vi "WaitForSpecificCommResponse.vi"(4 "CMD sent":string, 6 "Check period (msecs)":dbl=30.0, 7 "Display err mess?":bool=TRUE, 8 "error in (no error)":errorcluster, 9 "Timeout (mSecs)":dbl=3000.0, 10 "Wait for":string, 11 "VISA Refnum in":refnum<visa-resource-name>="COM30") -> (0 "error out":errorcluster, 1 "timeout":bool, 2 "Response":string, 3 "VISA Refnum out":refnum<visa-resource-name>, 5 "Elapsed secs":dbl)   [LabVIEW 2024]
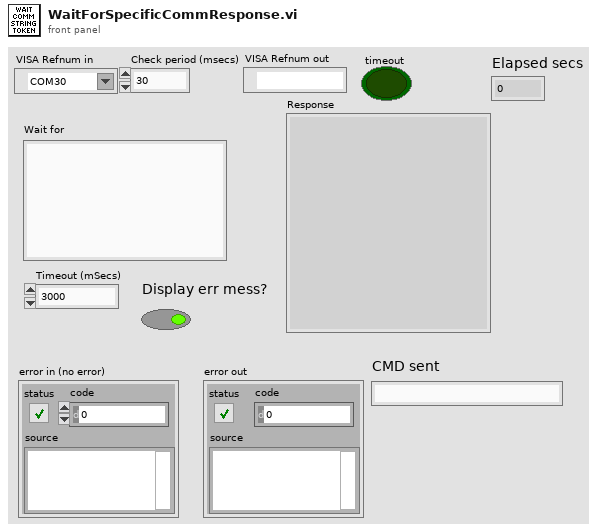
[diagram p1: front panel]
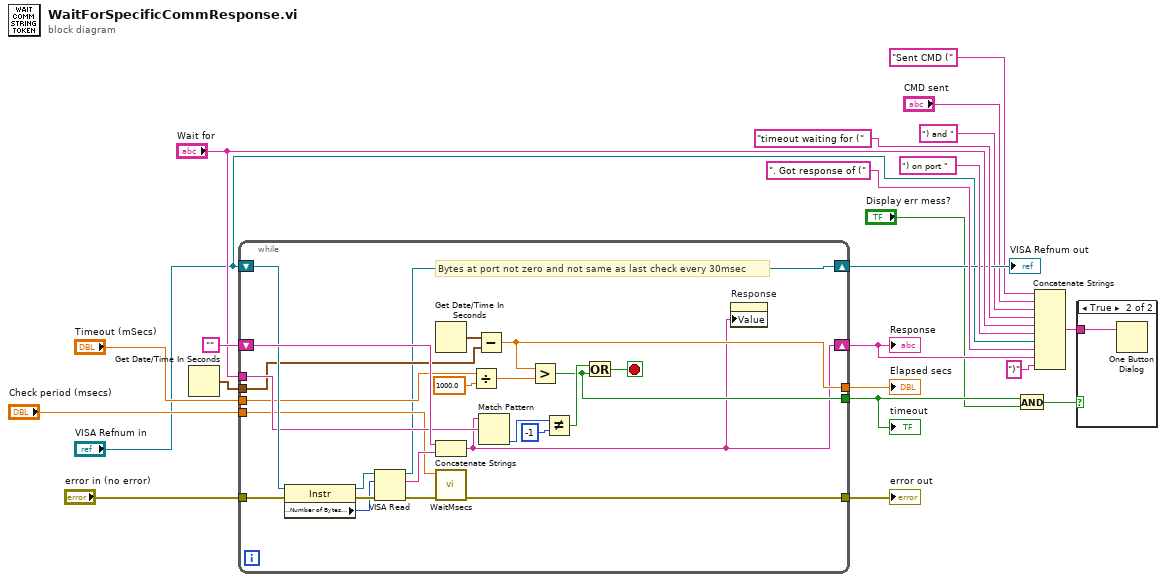
[diagram p0: block diagram]
diagram:
  n1 = Get Date/Time In Seconds() -> (seconds since 1Jan1904=w19:timestamp)
  n2 = while {
    shift-right: [w23] -> w14
    shift-left: "" -> [w43]
    tunnel: "error in (no error)" -> [w38]
    tunnel: "Wait for" -> [w37]
    tunnel: [w35] -> w21
    tunnel: [w27] -> w7
    tunnel: "Timeout (mSecs)" -> [w33]
    tunnel: "Check period (msecs)" -> [w31]
    tunnel: w19 -> [w29]
    shift-right: [w25] -> w11
    shift-left: "VISA Refnum in" -> [w39]
    tunnel: [w24] -> w1
    stop <- w34 stop-if-true
    # "Bytes at port not zero and not same as last check every 30msec"
    n3 = property class="Instr"(reference=w39, error in=w38) -> (reference out=w44:refnum<visa-resource-name>, error out=w46:errorcluster, "Serial Settings:Number of Bytes at Serial Port"=w45:u32)
    n4 = VISA Read(VISA resource name=w44, byte count=w45, error in (no error)=w46) -> (VISA resource name out=w25:refnum<visa-resource-name>, read buffer=w42:string, error out=w36:errorcluster)  [unwired: 1 out]
    n5 = Get Date/Time In Seconds() -> (seconds since 1Jan1904=w30:timestamp)
    n6 = Concatenate Strings(w43, w42) -> (w23:string)
    n7 = call "WaitMsecs.vi"("error in (no error)"=w36, "Wait Msecs"=w31) -> ("error out"=w35:errorcluster)  [unwired: 9 in]
    n8 = Divide(x=w33, y=1000.0) -> (x/y=w28:dbl)
    n9 = Subtract(x=w30, y=w29) -> (x-y=w24:dbl)
    n10 = Match Pattern(string=w23, regular expression=w37) -> (offset past match=w41:i32)  [unwired: 1 in, 3 out]
    n11 = Greater?(x=w24, y=w28) -> (0:w27:bool)
    n12 = Not Equal?(x=w41, y=-1) -> (x != y?=w32:bool)
    n13 = Or(x=w32, y=w27) -> (x .or. y?=w34:bool)
    n14 = property on="Response" class="Str"("Value"=w23) -> ()  [unwired: 2 in, 2 out]
  }
  "error out" <- w21
  "timeout" <- w7
  "VISA Refnum out" <- w11
  "Response" <- w14
  "Elapsed secs" <- w1
  n15 = And(x=w7, y="Display err mess?") -> (x .and. y?=w5:bool)
  n16 = Concatenate Strings("Sent CMD (" ("string"), "CMD sent", ") and " ("string"), "timeout waiting for (" ("string"), "Wait for", ") on port " ("string"), "VISA Refnum in", ". Got response of (" ("string"), w14, ")" ("string")) -> (w12:string)
  n17 = case shown="True" w5 {
    tunnel: w12 -> [_ w47]
    frame False {
    }
    frame True {
      n18 = One Button Dialog(message=w47) -> ()  [unwired: 1 in, 1 out]
    }
  }
